vi "CRYAlignment Harmonic curves.vi"(6 "Harmonics order":dbl[](array[numeric]), 7 "HT Option":bool[](array[boolean]), 8 "Std Error":dbl, 9 "Total Noise":cluster{"x":dbl, "y":dbl, "z":dbl}[](array[cluster]), 10 "Standard Error":cluster{cluster{"x":dbl, "y":dbl, "z":dbl}[]}[](array[cluster]), 11 "Harmonic Curves":cluster{cluster{"x":dbl, "y":dbl, "z":dbl}[]}[](array[cluster])) -> (3 "Freq Curves Out":cluster{cluster{"x":dbl, "y":dbl, "z":dbl}[]}[](array[cluster]))   [LabVIEW 2013]
panel:
  # "* measurement confidence\n0. Standard Error\n1. Confidence Limits\n2. Total Noise\n\n*Harmonics\n3. Harmonics @meas.Frq\n4. Total Distortion\n5. THD [%]\n6. THD Normalized [%]\n7. THD + Noise [%]\n8. Rub & Buzz [%]\n9. Rub & Buzz Norm'd [%]\n10. Perceptual Rub & Buzz\n\nIM\n11. Total IM\n12. Total IM [%]\n13. Total IM + Noise [%]\n\nDiff\n14. Total Diff\n15. Total DFD [%]\n16. Total DFD + Noise [%]"
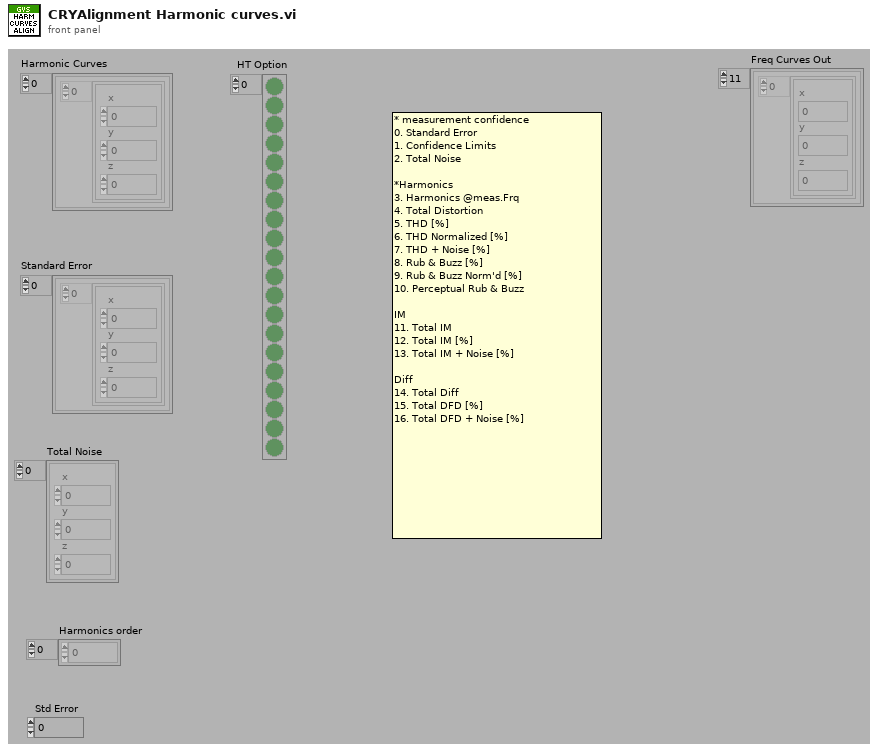
[diagram p1: front panel]
types:
  T1 = cluster{"Total Noise":cluster{"x":dbl, "y":dbl, "z":dbl}[]}
  T2 = cluster{"Total Noise":cluster{"x":dbl, "y":dbl, "z":dbl}[]}[]
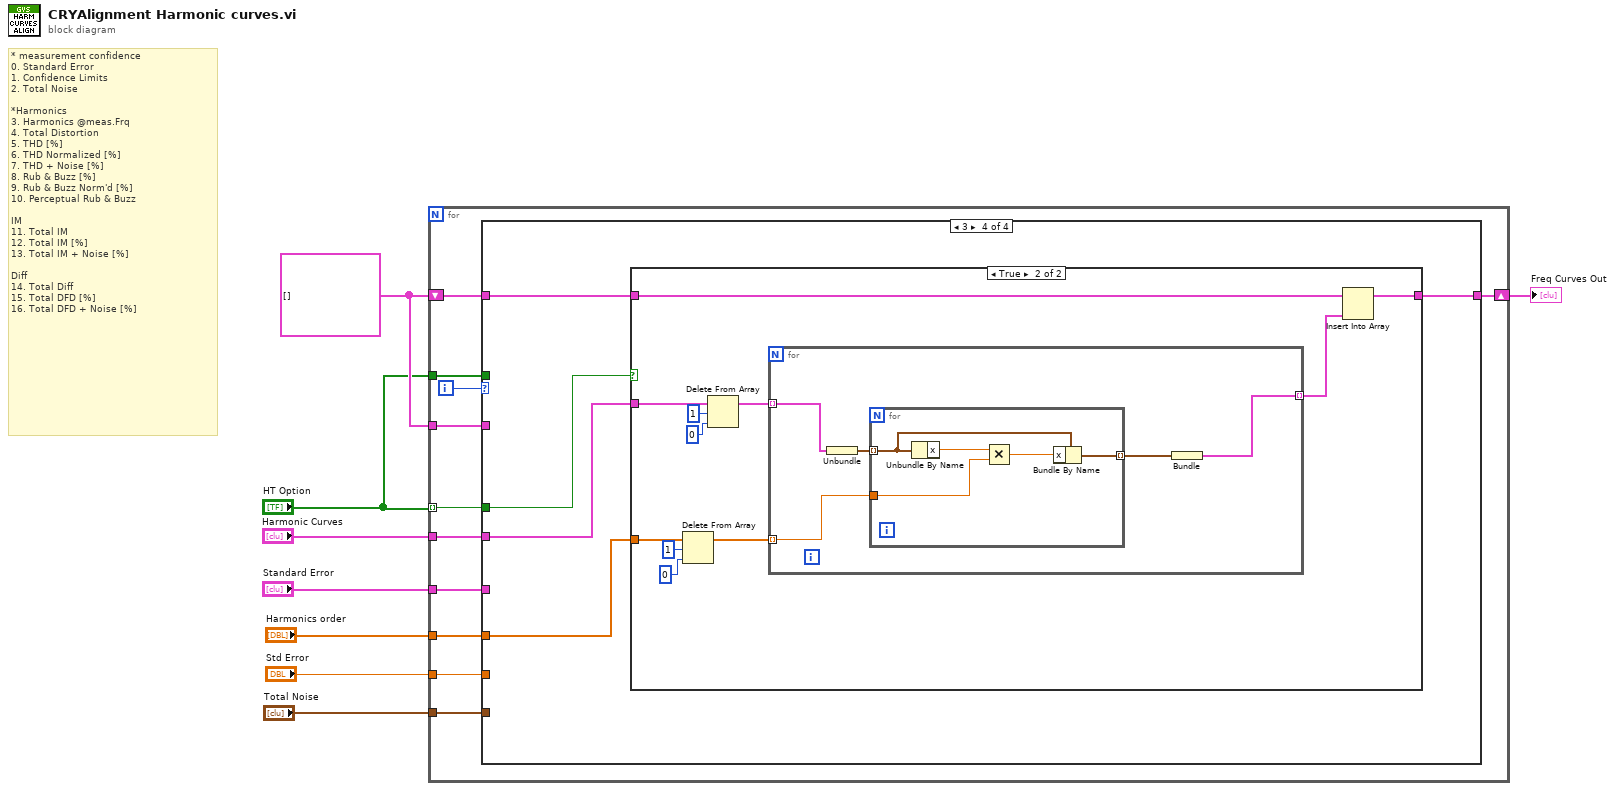
[diagram p0: block diagram]
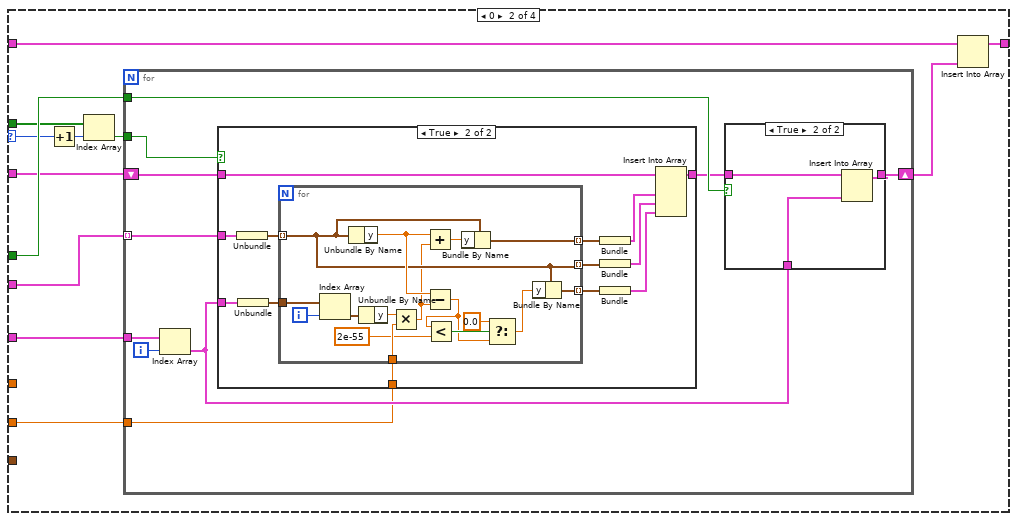
[diagram p3: hidden frame]
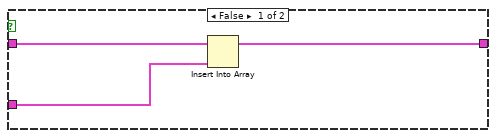
[diagram p5: hidden frame]
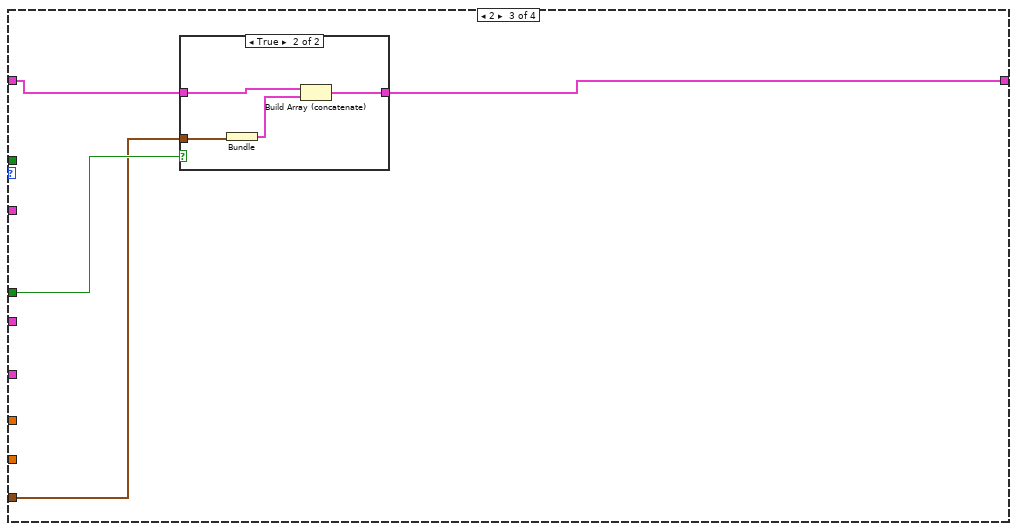
[diagram p6: hidden frame]
diagram:
  w8 = cluster{cluster{"x":dbl, "y":dbl, "z":dbl}[]}[] [] ("Freq resp curves clipped")
  # "* measurement confidence\n0. Standard Error\n1. Confidence Limits\n2. Total Noise\n\n*Harmonics\n3. Harmonics @meas.Frq\n4. Total Distortion\n5. THD [%]\n6. THD Normalized [%]\n7. THD + Noise [%]\n8. Rub & Buzz [%]\n9. Rub & Buzz Norm'd [%]\n10. Perceptual Rub & Buzz\n\nIM\n11. Total IM\n12. Total IM [%]\n13. Total IM + Noise [%]\n\nDiff\n14. Total Diff\n15. Total DFD [%]\n16. Total DFD + Noise [%]"
  n1 = for {
    tunnel: "HT Option" -> [w17] mode=indexing
    shift-right: [w18] -> w2
    shift-left: w8 -> [w19]
    tunnel: "Harmonic Curves" -> [w15]
    tunnel: "HT Option" -> [w14]
    tunnel: "Standard Error" -> [w13]
    tunnel: w8 -> [w12]
    tunnel: "Harmonics order" -> [w11]
    tunnel: "Total Noise" -> [w10]
    tunnel: "Std Error" -> [w9]
    i -> [w16]
    n2 = case shown="3" w16 {
      selector: w16 -> [_ w29 _ _]
      tunnel: w19 -> [w20 w24 w82 w90]
      tunnel: [w20 w25 w81 w89] -> w18
      tunnel: w17 -> [_ w31 w80 w92]
      tunnel: w15 -> [_ w32 _ w91]
      tunnel: w14 -> [_ w30 _ _]
      tunnel: w13 -> [_ w26 _ _]
      tunnel: w12 -> [_ w22 _ _]
      tunnel: w11 -> [_ _ _ w88]
      tunnel: w10 -> [_ _ w79 _]
      tunnel: w9 -> [_ w21 _ _]
      frame Default {
      }
      frame 0 {
        n3 = Increment(x=w29) -> (x+1=w28:i32)
        n4 = Index Array(array=w30, index=w28) -> (element=w27:bool)
        n5 = for {
          tunnel: w32 -> [w37] mode=indexing
          tunnel: w27 -> [w40]
          shift-right: [w41] -> w23
          shift-left: w22 -> [w42]
          tunnel: w31 -> [w39]
          tunnel: w26 -> [w36]
          tunnel: w21 -> [w33]
          i -> [w35]
          n6 = Index Array(array=w36, index=w35) -> (element=w34:cluster{cluster{"x":dbl, "y":dbl, "z":dbl}[]})
          n7 = case shown="True" w40 {
            tunnel: w37 -> [w47 w59]
            tunnel: w42 -> [w49 w62]
            tunnel: [w48 w61] -> w38
            tunnel: w34 -> [_ w60]
            tunnel: w33 -> [_ w56]
            frame False {
              n8 = Insert Into Array(array=w49, new element=w47) -> (w48:cluster{cluster{"x":dbl, "y":dbl, "z":dbl}[]}[])  [unwired: 1 in]
            }
            frame True {
              n9 = Unbundle(w59) -> (w54:cluster{"x":dbl, "y":dbl, "z":dbl}[])
              n10 = Unbundle(w60) -> (w53:cluster{"x":dbl, "y":dbl, "z":dbl}[])
              n11 = for {
                tunnel: w53 -> [w65]
                tunnel: w54 -> [w75] mode=indexing
                tunnel: [w73] -> w52 mode=indexing
                tunnel: [w75] -> w51 mode=indexing
                tunnel: [w76] -> w50 mode=indexing
                tunnel: w56 -> [w74]
                i -> [w63]
                n12 = Index Array(array=w65, index=w63) -> (element=w64:cluster{"x":dbl, "y":dbl, "z":dbl})
                n13 = Unbundle By Name(w75) -> ("y"=w77:dbl)
                n14 = Unbundle By Name(w64) -> ("y"=w71:dbl)
                n15 = Multiply(x=w71, y=w74) -> (x*y=w72:dbl)
                n16 = Add(x=w77, y=w72) -> (x+y=w78:dbl)
                n17 = Subtract(x=w77, y=w72) -> (x-y=w68:dbl)
                n18 = Less?(x=w68, y=2e-55 ("t")) -> (x < y?=w70:bool)
                n19 = Bundle By Name(cluster=w75, "y"=w78) -> (w73:cluster{"x":dbl, "y":dbl, "z":dbl})
                n20 = Select(t=0.0, s=w70, f=w68) -> (s? t:f=w67:dbl)
                n21 = Bundle By Name(cluster=w75, "y"=w67) -> (w76:cluster{"x":dbl, "y":dbl, "z":dbl})
              }
              n22 = Bundle(w52) -> (w58:cluster{cluster{"x":dbl, "y":dbl, "z":dbl}[]})  [unwired: 1 in]
              n23 = Bundle(w51) -> (w57:cluster{cluster{"x":dbl, "y":dbl, "z":dbl}[]})  [unwired: 1 in]
              n24 = Bundle(w50) -> (w55:cluster{cluster{"x":dbl, "y":dbl, "z":dbl}[]})  [unwired: 1 in]
              n25 = Insert Into Array(array=w62, new element #1=w58, new element #2=w57, new element #3=w55) -> (w61:cluster{cluster{"x":dbl, "y":dbl, "z":dbl}[]}[])  [unwired: 1 in]
            }
          }
          n26 = case shown="True" w39 {
            tunnel: w38 -> [w43 w46]
            tunnel: [w43 w45] -> w41
            tunnel: w34 -> [_ w44]
            frame False {
            }
            frame True {
              n27 = Insert Into Array(array=w46, new element=w44) -> (w45:cluster{cluster{"x":dbl, "y":dbl, "z":dbl}[]}[])  [unwired: 1 in]
            }
          }
        }
        n28 = Insert Into Array(array=w24, new element=w23) -> (w25:cluster{cluster{"x":dbl, "y":dbl, "z":dbl}[]}[])  [unwired: 1 in]
      }
      frame 2 {
        n29 = case shown="True" w80 {
          tunnel: w82 -> [w83 w87]
          tunnel: w79 -> [_ w85]
          tunnel: [w83 w86] -> w81
          frame False {
          }
          frame True {
            n30 = Bundle("Total Noise"=w85) -> (w84:T1)  [unwired: 1 in]
            n31 = Build Array (concatenate)(w87, w84) -> (w86:T2)
          }
        }
      }
      frame 3 {
        n32 = case shown="True" w92 {
          tunnel: w91 -> [_ w95]
          tunnel: w90 -> [w93 w104]
          tunnel: [w93 w102] -> w89
          tunnel: w88 -> [_ w101]
          frame False {
          }
          frame True {
            n33 = Delete From Array(array=w101, length=1, index=0) -> (array with subset deleted=w98:dbl[])  [unwired: 1 out]
            n34 = Delete From Array(array=w95, length=1, index=0) -> (array with subset deleted=w94:cluster{cluster{"x":dbl, "y":dbl, "z":dbl}[]}[])  [unwired: 1 out]
            n35 = for {
              tunnel: [w105] -> w103 mode=indexing
              tunnel: w98 -> [w107] mode=indexing
              tunnel: w94 -> [w108] mode=indexing
              n36 = Unbundle(w108) -> (w109:cluster{"x":dbl, "y":dbl, "z":dbl}[])
              n37 = for {
                tunnel: w109 -> [w114] mode=indexing
                tunnel: w107 -> [w112]
                tunnel: [w110] -> w106 mode=indexing
                n38 = Unbundle By Name(w114) -> ("x"=w113:dbl)
                n39 = Multiply(x=w113, y=w112) -> (x*y=w111:dbl)
                n40 = Bundle By Name(cluster=w114, "x"=w111) -> (w110:cluster{"x":dbl, "y":dbl, "z":dbl})
              }
              n41 = Bundle(w106) -> (w105:cluster{cluster{"x":dbl, "y":dbl, "z":dbl}[]})  [unwired: 1 in]
            }
            n42 = Insert Into Array(array=w104, new element=w103) -> (w102:cluster{cluster{"x":dbl, "y":dbl, "z":dbl}[]}[])  [unwired: 1 in]
          }
        }
      }
    }
  }
  "Freq Curves Out" <- w2
